vi "Step Core.vi"(8 "error in (no error)":errorcluster, 11 "Generic DUT Setup in":refnum<class "Generic DUT Setup.lvclass">) -> (0 "error out":errorcluster, 3 "Generic DUT Setup out":refnum<class "Generic DUT Setup.lvclass">)   [LabVIEW 2018, in "Generic DUT Setup.lvlib" / "Generic DUT Setup.lvclass"]
uses:
  Generic DUT Setup.lvclass
  C:/Sequence Automation/Plugins/Measurement Interface.lvlibp/Measurement Interface.lvclass
  Generic DUT Setup.lvclass/Generic DUT Setup.ctl
  Private Methods/Write Sequence Call Step.vi
  Private Methods/Read Sequence Call Step.vi
  Plugins/Measurement Interface.lvlibp/Private Methods/Sequence Call Step/Read Sequence Call Step Dictionary.vi
  Plugins/Sequence Call Step Dictionary.lvlibp/Sequence Call Step Dictionary.lvclass
  Plugins/Measurement Interface.lvlibp/Measurement Interface.lvclass
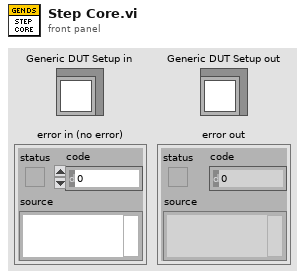
[diagram p1: front panel]
types:
  T1 = typedef "Sequence Call Step Dictionary.lvlibp/Sequence Call Step Dictionary.lvclass/Sequence Call Step.ctl" = cluster{"Sequence Call Step Reference":refnum<k7>, "Sequence Call Parameters":T2[]}
  T2 = typedef "Sequence Call Step Dictionary.lvlibp/Sequence Call Step Dictionary.lvclass/Parameter.ctl" = cluster{"Name":string, "PropertyObject Type":enum16{"Container", "String", "Boolean", "Number", "NamedType", "Reference", "Array", "Aperture Time"}}
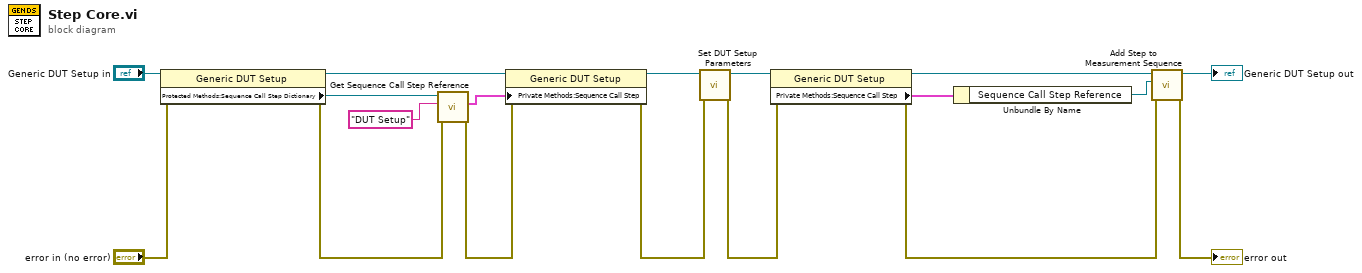
[diagram p0: block diagram]
diagram:
  n1 = property class="Generic DUT Setup"(reference="Generic DUT Setup in", error in="error in (no error)") -> (reference out=w11:refnum<class "Generic DUT Setup.lvclass">, error out=w15:errorcluster, "Protected Methods:Sequence Call Step Dictionary"=w16:refnum<class "Sequence Call Step Dictionary.lvclass">)
  n2 = call "Get Sequence Call Step Reference.vi"("error in (no error)"=w15, "Sequence Call to Retrieve"="DUT Setup", "Sequence Call Step Dict in"=w16) -> ("error out"=w14:errorcluster, "Sequence Call Step Out"=w10:T1)  [unwired: 6 in, 1 out]
  n3 = property class="Generic DUT Setup"(reference=w11, error in=w14, "Private Methods:Sequence Call Step"=w10) -> (reference out=w8:refnum<class "Generic DUT Setup.lvclass">, error out=w12:errorcluster)
  n4 = call "Set DUT Setup Parameters.vi"("error in (no error)"=w12, "Generic DUT Setup in"=w8) -> ("error out"=w9:errorcluster, "Generic DUT Setup out"=w4:refnum<class "Generic DUT Setup.lvclass">)  [unwired: 8 in]
  n5 = property class="Generic DUT Setup"(reference=w4, error in=w9) -> (reference out=w3:refnum<class "Generic DUT Setup.lvclass">, error out=w5:errorcluster, "Private Methods:Sequence Call Step"=w2:T1)
  n6 = Unbundle By Name(w2) -> ("Sequence Call Step Reference"=w1:refnum<k7>)
  n7 = call "Add Step to Measurement Sequence.vi"("error in (no error)"=w5, "Step to Add"=w1, "Measurement Interface in"=w3) -> ("error out"=→"error out":errorcluster, "Measurement Interface out"=→"Generic DUT Setup out":refnum<class "Generic DUT Setup.lvclass">)  [unwired: 7 in]
